vi "ep_Check Status Channel Validation.vi"(8 "error in (no error)":errorcluster, 11 "status channel info in":T1[](array[typedef])) -> (0 "error out":errorcluster, 3 "status channel info out":T1[](array[typedef]))   [LabVIEW 2011, in "NI_EP_COMTRADE.lvlib"]
uses:
  <vilib>/addons/Electrical Power/File IO/NI_EP_COMTRADE.lvlib
  <vilib>/addons/Electrical Power/File IO/COMTRADE/typedefs/ep_Status Channel Info (UI).ctl
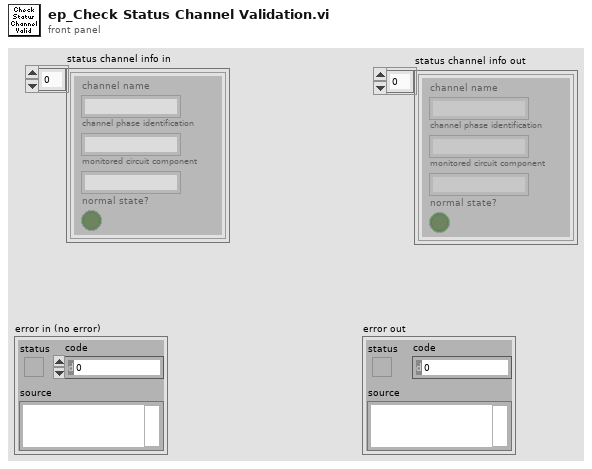
[diagram p1: front panel]
types:
  T1 = typedef "NI_EP_COMTRADE.lvlib/ep_Status Channel Info (UI).ctl" = cluster{"channel name":string, "channel phase identification":string, "monitored circuit component":string, "normal state?":bool}
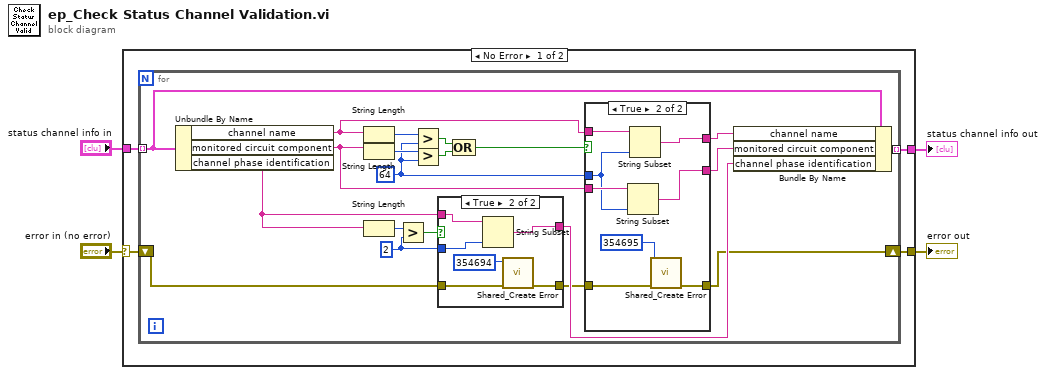
[diagram p0: block diagram]
diagram:
  n1 = case shown="No Error" "error in (no error)" {
    selector: "error in (no error)" -> [w7 w49]
    tunnel: [w6 w49] -> w3
    tunnel: "status channel info in" -> [w8 w48]
    tunnel: [w5 w48] -> w1
    frame No Error {
      n2 = for {
        tunnel: w8 -> [w20] mode=indexing
        shift-right: [w9] -> w6
        shift-left: w7 -> [w21]
        tunnel: [w18] -> w5 mode=indexing
        w25 = 2 ("y")
        w14 = 64 ("y")
        n3 = Unbundle By Name(w20) -> ("channel name"=w15:string, "monitored circuit component"=w13:string, "channel phase identification"=w22:string)
        n4 = String Length(string=w15) -> (length=w24:i32)
        n5 = String Length(string=w13) -> (length=w28:i32)
        n6 = String Length(string=w22) -> (length=w26:i32)
        n7 = Greater?(x=w26, y=w25) -> (0:w10:bool)
        n8 = Greater?(x=w24, y=w14) -> (0:w23:bool)
        n9 = Greater?(x=w28, y=w14) -> (0:w27:bool)
        n10 = case shown="True" w10 {
          tunnel: w21 -> [w41 w44]
          tunnel: [w41 w43] -> w17
          tunnel: w22 -> [w40 w47]
          tunnel: w25 -> [_ w46]
          tunnel: [w40 w45] -> w19
          frame False {
          }
          frame True {
            n11 = String Subset(string=w47, length (rest)=w46) -> (substring=w45:string)  [unwired: 1 in]
            n12 = call <vilib>:"Shared_Create Error.vi"("error in (no error)"=w44, "error code (0)"=354694 ("code")) -> ("error out"=w43:errorcluster)  [unwired: 9 in]
          }
        }
        n13 = Compound Arithmetic op=OR(w23, w27) -> (w16:bool)
        n14 = case shown="True" w16 {
          tunnel: w15 -> [w31 w39]
          tunnel: w13 -> [w30 w38]
          tunnel: w14 -> [_ w37]
          tunnel: w17 -> [w29 w34]
          tunnel: [w31 w36] -> w12
          tunnel: [w30 w35] -> w11
          tunnel: [w29 w33] -> w9
          frame False {
          }
          frame True {
            n15 = String Subset(string=w38, length (rest)=w37) -> (substring=w35:string)  [unwired: 1 in]
            n16 = String Subset(string=w39, length (rest)=w37) -> (substring=w36:string)  [unwired: 1 in]
            n17 = call <vilib>:"Shared_Create Error.vi"("error in (no error)"=w34, "error code (0)"=354695 ("code")) -> ("error out"=w33:errorcluster)  [unwired: 9 in]
          }
        }
        n18 = Bundle By Name(cluster=w20, "channel name"=w12, "monitored circuit component"=w11, "channel phase identification"=w19) -> (w18:T1)
      }
    }
    frame Error {
    }
  }
  "error out" <- w3
  "status channel info out" <- w1
